vi "Assemble all modules.vi"(2 "Module List 2":T4(array[cluster])=[{"Enable"=TRUE, "Abs Start Time"="", "Module"=1, "String"="laser relock", "Array"=["A", "1"]}, {"Enable"=FALSE, "Abs Start Time"="", "Module"=0, "String"="", "Array"=["c", "7"]}, {"Enable"=TRUE, "Abs Start Time"="", "Module"=8, "String"="", "Array"=[]}, {"Enable"=TRUE, "Abs Start Time"="", "Module"=0, "String"="IP bias bleed on", "Array"=["B", "3"]}, {"Enable"=TRUE, "Abs Start Time"="", "Module"=0, "String"="IP master switch on", "Array"=["B", "2"]}, {"Enable"=FALSE, "Abs Start Time"="", "Module"=11, "String"="", "Array"=[]}, {"Enable"=FALSE, "Abs Start Time"="", "Module"=0, "String"="laser unlock for return", "Array"=["A", "1"]}, {"Enable"=FALSE, "Abs Start Time"="", "Module"=1, "String"="laser unlock for return", "Array"=["A", "1"]}, {"Enable"=FALSE, "Abs Start Time"="", "Module"=20, "String"="E/W shim for MOT", "Array"=["0", "0"]}, {"Enable"=FALSE, "Abs Start Time"="", "Module"=20, "String"="U/D shim for MOT", "Array"=["1", "-1"]}, {"Enable"=FALSE, "Abs Start Time"="", "Module"=20, "String"="N/S shim for MOT", "Array"=["2", "-1.5"]}, {"Enable"=FALSE, "Abs Start Time"="", "Module"=3, "String"="", "Array"=[]}] {"Module" items=["TTL high                                                                                 ", "TTL low                          ", "Camera Strobe                   ", "CMOT", "Defaults                           ", "Fluorescence pulse           ", "IP trap                         ", "Kinetics OD image          ", "Kinetics picture", "Kinetics probe pulse", "MOT light only                ", "MOT off                                   ", "MOT on                         ", "Move cart                      ", "OD image                     ", "Optical pumping          ", "Picture                             ", "Probe Pulse", "Quadrupole trap             ", "Quadrupole trap off", "QTrap off for OT        ", "Rb removal       ", "Molasses          ", "STIRAP", "OT B Field Off", "High field     ", "Utility Module 07     ", "Low Field", "Final B field ramps    ", "K removal    ", "Static DAC", "GPIB", "Molecule OD image", "Mol probe pulse", "Mol picture", "Unused OD image", "Unused probe pulse", "Unused picture", "K img repump", "STIRAP back 4 imaging", "B Field off", "Field Calibration", "Utility Module 15", "Utility Module 16", "Utility Module 17", "Utility Module 18", "Utility Module 19", "Utility Module 20"]}, 3 "durations":dbl[](array[numeric])=[0.0, 2400.0, 8635.078497322447, 3100.0, 1000.0, 2000.0] format="%.2f", 4 "Module List 6":T4(array[cluster])=[{"Enable"=TRUE, "Abs Start Time"="", "Module"=1, "String"="", "Array"=["c", "7"]}] {"Module" items=["TTL high                                                                                 ", "TTL low                          ", "Camera Strobe                   ", "CMOT", "Defaults                           ", "Fluorescence pulse           ", "IP trap                         ", "Kinetics OD image          ", "Kinetics picture", "Kinetics probe pulse", "MOT light only                ", "MOT off                                   ", "MOT on                         ", "Move cart                      ", "OD image                     ", "Optical pumping          ", "Picture                             ", "Probe Pulse", "Quadrupole trap             ", "Quadrupole trap off", "QTrap off for OT        ", "Rb removal       ", "Molasses          ", "STIRAP", "OT B Field Off", "High field     ", "Utility Module 07     ", "Low Field", "Final B field ramps    ", "K removal    ", "Static DAC", "GPIB", "Molecule OD image", "Mol probe pulse", "Mol picture", "Unused OD image", "Unused probe pulse", "Unused picture", "K img repump", "STIRAP back 4 imaging", "B Field off", "Field Calibration", "Utility Module 15", "Utility Module 16", "Utility Module 17", "Utility Module 18", "Utility Module 19", "Utility Module 20"]}, 5 "Module List 1":T4(array[cluster])=[{"Enable"=TRUE, "Abs Start Time"="", "Module"=0, "String"="dynamic DAC trigger", "Array"=["D", "14"]}, {"Enable"=TRUE, "Abs Start Time"="", "Module"=1, "String"="trigger down", "Array"=["D", "14"]}, {"Enable"=TRUE, "Abs Start Time"="", "Module"=19, "String"="", "Array"=[]}, {"Enable"=TRUE, "Abs Start Time"="", "Module"=20, "String"="K trap freq for CMOT", "Array"=["5", "4.6"]}, {"Enable"=TRUE, "Abs Start Time"="", "Module"=20, "String"="E/W shim for Qtrap loading", "Array"=["0", "-1"]}, {"Enable"=TRUE, "Abs Start Time"="", "Module"=20, "String"="U/D shim for Qtrap loading", "Array"=["1", "-1.5"]}, {"Enable"=TRUE, "Abs Start Time"="", "Module"=20, "String"="N/S shim for Qtrap loading", "Array"=["2", "-1"]}, {"Enable"=TRUE, "Abs Start Time"="", "Module"=20, "String"="repump K freq for OP", "Array"=["3", "0.05"]}, {"Enable"=TRUE, "Abs Start Time"="", "Module"=20, "String"="E/W shim for molasses 0", "Array"=["0", "-1"]}, {"Enable"=TRUE, "Abs Start Time"="", "Module"=20, "String"="U/D shim for molasses -0.6", "Array"=["1", "0.1"]}, {"Enable"=TRUE, "Abs Start Time"="", "Module"=20, "String"="N/S shim for molasses 0", "Array"=["2", "2"]}, {"Enable"=TRUE, "Abs Start Time"="", "Module"=8, "String"="", "Array"=["", ""]}, {"Enable"=TRUE, "Abs Start Time"="", "Module"=1, "String"="close Rb shutter(takes 1.4 ms", "Array"=["B", "0"]}, {"Enable"=FALSE, "Abs Start Time"="", "Module"=12, "String"="\n", "Array"=[]}, {"Enable"=FALSE, "Abs Start Time"="", "Module"=0, "String"="scope trigger", "Array"=["c", "7"]}, {"Enable"=FALSE, "Abs Start Time"="", "Module"=1, "String"="", "Array"=["c", "7"]}, {"Enable"=TRUE, "Abs Start Time"="", "Module"=14, "String"="", "Array"=[]}, {"Enable"=TRUE, "Abs Start Time"="", "Module"=20, "String"="K trap freq for MOT", "Array"=["5", "4.3"]}, {"Enable"=TRUE, "Abs Start Time"="", "Module"=20, "String"=" K repump freq for MOT freq", "Array"=["3", "0"]}, {"Enable"=TRUE, "Abs Start Time"="", "Module"=20, "String"="E/W shim for Qtrap", "Array"=["0", "2"]}, {"Enable"=TRUE, "Abs Start Time"="", "Module"=20, "String"="U/D shim for Qtrap", "Array"=["1", "2"]}, {"Enable"=TRUE, "Abs Start Time"="", "Module"=20, "String"="N/S shim for Qtrap", "Array"=["2", "2"]}, {"Enable"=TRUE, "Abs Start Time"="", "Module"=10, "String"="", "Array"=["-10"]}, {"Enable"=TRUE, "Abs Start Time"="", "Module"=0, "String"="laser unlock", "Array"=["A", "1"]}] {"Module" items=["TTL high                                                                                 ", "TTL low                          ", "Camera Strobe                   ", "CMOT", "Defaults                           ", "Fluorescence pulse           ", "IP trap                         ", "Kinetics OD image          ", "Kinetics picture", "Kinetics probe pulse", "MOT light only                ", "MOT off                                   ", "MOT on                         ", "Move cart                      ", "OD image                     ", "Optical pumping          ", "Picture                             ", "Probe Pulse", "Quadrupole trap             ", "Quadrupole trap off", "QTrap off for OT        ", "Rb removal       ", "Molasses          ", "STIRAP", "OT B Field Off", "High field     ", "Utility Module 07     ", "Low Field", "Final B field ramps    ", "K removal    ", "Static DAC", "GPIB", "Molecule OD image", "Mol probe pulse", "Mol picture", "Unused OD image", "Unused probe pulse", "Unused picture", "K img repump", "STIRAP back 4 imaging", "B Field off", "Field Calibration", "Utility Module 15", "Utility Module 16", "Utility Module 17", "Utility Module 18", "Utility Module 19", "Utility Module 20"]}, 6 "Module List 5":T4(array[cluster])=[{"Enable"=TRUE, "Abs Start Time"="", "Module"=0, "String"="", "Array"=["c", "7"]}] {"Module" items=["TTL high                                                                                 ", "TTL low                          ", "Camera Strobe                   ", "CMOT", "Defaults                           ", "Fluorescence pulse           ", "IP trap                         ", "Kinetics OD image          ", "Kinetics picture", "Kinetics probe pulse", "MOT light only                ", "MOT off                                   ", "MOT on                         ", "Move cart                      ", "OD image                     ", "Optical pumping          ", "Picture                             ", "Probe Pulse", "Quadrupole trap             ", "Quadrupole trap off", "QTrap off for OT        ", "Rb removal       ", "Molasses          ", "STIRAP", "OT B Field Off", "High field     ", "Utility Module 07     ", "Low Field", "Final B field ramps    ", "K removal    ", "Static DAC", "GPIB", "Molecule OD image", "Mol probe pulse", "Mol picture", "Unused OD image", "Unused probe pulse", "Unused picture", "K img repump", "STIRAP back 4 imaging", "B Field off", "Field Calibration", "Utility Module 15", "Utility Module 16", "Utility Module 17", "Utility Module 18", "Utility Module 19", "Utility Module 20"]}, 7 "Module List 4":T4(array[cluster])=[{"Enable"=TRUE, "Abs Start Time"="", "Module"=1, "String"="IP master switch off", "Array"=["B", "2"]}, {"Enable"=TRUE, "Abs Start Time"="", "Module"=0, "String"="trigger scope", "Array"=["c", "7"]}, {"Enable"=TRUE, "Abs Start Time"="", "Module"=11, "String"="", "Array"=[]}, {"Enable"=TRUE, "Abs Start Time"="", "Module"=0, "String"="laser unlock for cart return", "Array"=["A", "1"]}, {"Enable"=TRUE, "Abs Start Time"="", "Module"=1, "String"="laser relock", "Array"=["A", "1"]}, {"Enable"=TRUE, "Abs Start Time"="", "Module"=20, "String"="E/W shim for MOT", "Array"=["0", "0"]}, {"Enable"=TRUE, "Abs Start Time"="", "Module"=20, "String"="U/D shim for MOT", "Array"=["1", "-1"]}, {"Enable"=TRUE, "Abs Start Time"="", "Module"=20, "String"="N/S shim for MOT", "Array"=["2", "-1.5"]}, {"Enable"=TRUE, "Abs Start Time"="", "Module"=3, "String"="", "Array"=[]}, {"Enable"=FALSE, "Abs Start Time"="", "Module"=3, "String"="", "Array"=[]}] {"Module" items=["TTL high                                                                                 ", "TTL low                          ", "Camera Strobe                   ", "CMOT", "Defaults                           ", "Fluorescence pulse           ", "IP trap                         ", "Kinetics OD image          ", "Kinetics picture", "Kinetics probe pulse", "MOT light only                ", "MOT off                                   ", "MOT on                         ", "Move cart                      ", "OD image                     ", "Optical pumping          ", "Picture                             ", "Probe Pulse", "Quadrupole trap             ", "Quadrupole trap off", "QTrap off for OT        ", "Rb removal       ", "Molasses          ", "STIRAP", "OT B Field Off", "High field     ", "Utility Module 07     ", "Low Field", "Final B field ramps    ", "K removal    ", "Static DAC", "GPIB", "Molecule OD image", "Mol probe pulse", "Mol picture", "Unused OD image", "Unused probe pulse", "Unused picture", "K img repump", "STIRAP back 4 imaging", "B Field off", "Field Calibration", "Utility Module 15", "Utility Module 16", "Utility Module 17", "Utility Module 18", "Utility Module 19", "Utility Module 20"]}, 8 "Module List 3":T4(array[cluster])=[{"Enable"=FALSE, "Abs Start Time"="", "Module"=0, "String"="", "Array"=[]}] {"Module" items=["TTL high                                                                                 ", "TTL low                          ", "Camera Strobe                   ", "CMOT", "Defaults                           ", "Fluorescence pulse           ", "IP trap                         ", "Kinetics OD image          ", "Kinetics picture", "Kinetics probe pulse", "MOT light only                ", "MOT off                                   ", "MOT on                         ", "Move cart                      ", "OD image                     ", "Optical pumping          ", "Picture                             ", "Probe Pulse", "Quadrupole trap             ", "Quadrupole trap off", "QTrap off for OT        ", "Rb removal       ", "Molasses          ", "STIRAP", "OT B Field Off", "High field     ", "Utility Module 07     ", "Low Field", "Final B field ramps    ", "K removal    ", "Static DAC", "GPIB", "Molecule OD image", "Mol probe pulse", "Mol picture", "Unused OD image", "Unused probe pulse", "Unused picture", "K img repump", "STIRAP back 4 imaging", "B Field off", "Field Calibration", "Utility Module 15", "Utility Module 16", "Utility Module 17", "Utility Module 18", "Utility Module 19", "Utility Module 20"]}, 9 "Module Enabled Array":bool[](array[boolean])=[TRUE, TRUE, TRUE, TRUE, TRUE, TRUE]) -> (0 "Saveit Array":T2(array[cluster])=[{"Cluster"={"Enable"=TRUE, "Abs Start Time"=0.1, "Module"=0, "String"="dynamic DAC trigger", "Array"=["D", "14"]}, "Ring"=0}, {"Cluster"={"Enable"=TRUE, "Abs Start Time"=10.0, "Module"=1, "String"="trigger down", "Array"=["D", "14"]}, "Ring"=0}, {"Cluster"={"Enable"=TRUE, "Abs Start Time"=947.0, "Module"=19, "String"="", "Array"=[]}, "Ring"=0}, {"Cluster"={"Enable"=TRUE, "Abs Start Time"=947.0, "Module"=20, "String"="K trap freq for CMOT", "Array"=["5", "4.6"]}, "Ring"=0}, {"Cluster"={"Enable"=TRUE, "Abs Start Time"=947.0, "Module"=20, "String"="E/W shim for Qtrap loading", "Array"=["0", "-1"]}, "Ring"=0}, {"Cluster"={"Enable"=TRUE, "Abs Start Time"=947.0, "Module"=20, "String"="U/D shim for Qtrap loading", "Array"=["1", "-1.5"]}, "Ring"=0}, {"Cluster"={"Enable"=TRUE, "Abs Start Time"=947.0, "Module"=20, "String"="N/S shim for Qtrap loading", "Array"=["2", "-1"]}, "Ring"=0}, {"Cluster"={"Enable"=TRUE, "Abs Start Time"=947.0, "Module"=20, "String"="repump K freq for OP", "Array"=["3", "0.05"]}, "Ring"=0}, {"Cluster"={"Enable"=TRUE, "Abs Start Time"=994.5, "Module"=20, "String"="E/W shim for molasses 0", "Array"=["0", "-1"]}, "Ring"=0}, {"Cluster"={"Enable"=TRUE, "Abs Start Time"=994.5, "Module"=20, "String"="U/D shim for molasses -0.6", "Array"=["1", "0.1"]}, "Ring"=0}, {"Cluster"={"Enable"=TRUE, "Abs Start Time"=994.5, "Module"=20, "String"="N/S shim for molasses 0", "Array"=["2", "2"]}, "Ring"=0}, {"Cluster"={"Enable"=TRUE, "Abs Start Time"=995.5, "Module"=8, "String"="", "Array"=["", ""]}, "Ring"=0}, {"Cluster"={"Enable"=TRUE, "Abs Start Time"=997.1, "Module"=1, "String"="close Rb shutter(takes 1.4 ms", "Array"=["B", "0"]}, "Ring"=0}, {"Cluster"={"Enable"=FALSE, "Abs Start Time"=998.5, "Module"=12, "String"="\n", "Array"=[]}, "Ring"=0}, {"Cluster"={"Enable"=FALSE, "Abs Start Time"=998.5, "Module"=0, "String"="scope trigger", "Array"=["c", "7"]}, "Ring"=0}, {"Cluster"={"Enable"=FALSE, "Abs Start Time"=999.0, "Module"=1, "String"="", "Array"=["c", "7"]}, "Ring"=0}, {"Cluster"={"Enable"=TRUE, "Abs Start Time"=1000.0, "Module"=14, "String"="", "Array"=[]}, "Ring"=0}, {"Cluster"={"Enable"=TRUE, "Abs Start Time"=1000.0, "Module"=20, "String"="K trap freq for MOT", "Array"=["5", "4.3"]}, "Ring"=0}, {"Cluster"={"Enable"=TRUE, "Abs Start Time"=1000.0, "Module"=20, "String"=" K repump freq for MOT freq", "Array"=["3", "0"]}, "Ring"=0}, {"Cluster"={"Enable"=TRUE, "Abs Start Time"=1000.0, "Module"=20, "String"="E/W shim for Qtrap", "Array"=["0", "2"]}, "Ring"=0}, {"Cluster"={"Enable"=TRUE, "Abs Start Time"=1000.0, "Module"=20, "String"="U/D shim for Qtrap", "Array"=["1", "2"]}, "Ring"=0}, {"Cluster"={"Enable"=TRUE, "Abs Start Time"=1000.0, "Module"=20, "String"="N/S shim for Qtrap", "Array"=["2", "2"]}, "Ring"=0}, {"Cluster"={"Enable"=TRUE, "Abs Start Time"=1000.0, "Module"=10, "String"="", "Array"=["-10"]}, "Ring"=0}, {"Cluster"={"Enable"=TRUE, "Abs Start Time"=1000.0, "Module"=0, "String"="laser unlock", "Array"=["A", "1"]}, "Ring"=0}, {"Cluster"={"Enable"=TRUE, "Abs Start Time"=0.0, "Module"=1, "String"="laser relock", "Array"=["A", "1"]}, "Ring"=1}, {"Cluster"={"Enable"=FALSE, "Abs Start Time"=500.0, "Module"=0, "String"="", "Array"=["c", "7"]}, "Ring"=1}, {"Cluster"={"Enable"=TRUE, "Abs Start Time"=500.0, "Module"=8, "String"="", "Array"=[]}, "Ring"=1}, {"Cluster"={"Enable"=TRUE, "Abs Start Time"=400.0, "Module"=0, "String"="IP bias bleed on", "Array"=["B", "3"]}, "Ring"=1}, {"Cluster"={"Enable"=TRUE, "Abs Start Time"=500.0, "Module"=0, "String"="IP master switch on", "Array"=["B", "2"]}, "Ring"=1}, {"Cluster"={"Enable"=FALSE, "Abs Start Time"=505.0, "Module"=11, "String"="", "Array"=[]}, "Ring"=1}, {"Cluster"={"Enable"=FALSE, "Abs Start Time"=2000.0, "Module"=0, "String"="laser unlock for return", "Array"=["A", "1"]}, "Ring"=1}, {"Cluster"={"Enable"=FALSE, "Abs Start Time"=3500.0, "Module"=1, "String"="laser unlock for return", "Array"=["A", "1"]}, "Ring"=1}, {"Cluster"={"Enable"=FALSE, "Abs Start Time"=3600.0, "Module"=20, "String"="E/W shim for MOT", "Array"=["0", "0"]}, "Ring"=1}, {"Cluster"={"Enable"=FALSE, "Abs Start Time"=3600.0, "Module"=20, "String"="U/D shim for MOT", "Array"=["1", "-1"]}, "Ring"=1}, {"Cluster"={"Enable"=FALSE, "Abs Start Time"=3600.0, "Module"=20, "String"="N/S shim for MOT", "Array"=["2", "-1.5"]}, "Ring"=1}, {"Cluster"={"Enable"=FALSE, "Abs Start Time"=18500.0, "Module"=3, "String"="", "Array"=[]}, "Ring"=1}, {"Cluster"={"Enable"=FALSE, "Abs Start Time"=0.0, "Module"=0, "String"="", "Array"=[]}, "Ring"=2}, {"Cluster"={"Enable"=TRUE, "Abs Start Time"=0.0, "Module"=1, "String"="IP master switch off", "Array"=["B", "2"]}, "Ring"=3}, {"Cluster"={"Enable"=TRUE, "Abs Start Time"=0.0, "Module"=0, "String"="trigger scope", "Array"=["c", "7"]}, "Ring"=3}, {"Cluster"={"Enable"=TRUE, "Abs Start Time"=5.0, "Module"=11, "String"="", "Array"=[]}, "Ring"=3}, {"Cluster"={"Enable"=TRUE, "Abs Start Time"=1500.0, "Module"=0, "String"="laser unlock for cart return", "Array"=["A", "1"]}, "Ring"=3}, {"Cluster"={"Enable"=TRUE, "Abs Start Time"=3000.0, "Module"=1, "String"="laser relock", "Array"=["A", "1"]}, "Ring"=3}, {"Cluster"={"Enable"=TRUE, "Abs Start Time"=3000.0, "Module"=20, "String"="E/W shim for MOT", "Array"=["0", "0"]}, "Ring"=3}, {"Cluster"={"Enable"=TRUE, "Abs Start Time"=3000.0, "Module"=20, "String"="U/D shim for MOT", "Array"=["1", "-1"]}, "Ring"=3}, {"Cluster"={"Enable"=TRUE, "Abs Start Time"=3000.0, "Module"=20, "String"="N/S shim for MOT", "Array"=["2", "-1.5"]}, "Ring"=3}, {"Cluster"={"Enable"=TRUE, "Abs Start Time"=3100.0, "Module"=3, "String"="", "Array"=[]}, "Ring"=3}, {"Cluster"={"Enable"=FALSE, "Abs Start Time"=18000.0, "Module"=3, "String"="", "Array"=[]}, "Ring"=3}, {"Cluster"={"Enable"=TRUE, "Abs Start Time"=0.0, "Module"=0, "String"="", "Array"=["c", "7"]}, "Ring"=4}, {"Cluster"={"Enable"=TRUE, "Abs Start Time"=200.0, "Module"=1, "String"="", "Array"=["c", "7"]}, "Ring"=5}] {"Ring" items=["TTL high                                                                                 ", "TTL low                          ", "Camera Strobe                   ", "Defaults                           ", "Fluorescence pulse           ", "IP trap                         ", "Kinetics OD image          ", "MOT light only                ", "MOT off                                   ", "MOT on                         ", "Move cart                      ", "OD image                     ", "Optical pumping          ", "Picture                             ", "Quadrupole trap             ", "Utility Module 01          ", "Utility Module 02           ", "Utility Module 03           ", "Utility Module 04           ", "CMOT", "Static DAQ", "GPIB"]; "Cluster"."Module" items=["TTL high                                                                                 ", "TTL low                          ", "Camera Strobe                   ", "CMOT", "Defaults                           ", "Fluorescence pulse           ", "IP trap                         ", "Kinetics OD image          ", "Kinetics picture", "Kinetics probe pulse", "MOT light only                ", "MOT off                                   ", "MOT on                         ", "Move cart                      ", "OD image                     ", "Optical pumping          ", "Picture                             ", "Probe Pulse", "Quadrupole trap             ", "Quadrupole trap off", "QTrap off for OT        ", "Rb removal       ", "Molasses          ", "STIRAP", "OT B Field Off", "High field     ", "Utility Module 07     ", "Low Field", "Final B field ramps    ", "K removal    ", "Static DAC", "GPIB", "Molecule OD image", "Mol probe pulse", "Mol picture", "Unused OD image", "Unused probe pulse", "Unused picture", "K img repump", "STIRAP back 4 imaging", "B Field off", "Field Calibration", "Utility Module 15", "Utility Module 16", "Utility Module 17", "Utility Module 18", "Utility Module 19", "Utility Module 20"]; "Cluster"."Abs Start Time" format="%.3f"}, 1 "Module Array":T1(array[cluster])=[{"Enable"=TRUE, "Abs Start Time"=0.1, "Module"=0, "String"="dynamic DAC trigger", "Array"=["D", "14"]}, {"Enable"=TRUE, "Abs Start Time"=10.0, "Module"=1, "String"="trigger down", "Array"=["D", "14"]}, {"Enable"=TRUE, "Abs Start Time"=947.0, "Module"=19, "String"="", "Array"=[]}, {"Enable"=TRUE, "Abs Start Time"=947.0, "Module"=20, "String"="K trap freq for CMOT", "Array"=["5", "4.6"]}, {"Enable"=TRUE, "Abs Start Time"=947.0, "Module"=20, "String"="E/W shim for Qtrap loading", "Array"=["0", "-1"]}, {"Enable"=TRUE, "Abs Start Time"=947.0, "Module"=20, "String"="U/D shim for Qtrap loading", "Array"=["1", "-1.5"]}, {"Enable"=TRUE, "Abs Start Time"=947.0, "Module"=20, "String"="N/S shim for Qtrap loading", "Array"=["2", "-1"]}, {"Enable"=TRUE, "Abs Start Time"=947.0, "Module"=20, "String"="repump K freq for OP", "Array"=["3", "0.05"]}, {"Enable"=TRUE, "Abs Start Time"=994.5, "Module"=20, "String"="E/W shim for molasses 0", "Array"=["0", "-1"]}, {"Enable"=TRUE, "Abs Start Time"=994.5, "Module"=20, "String"="U/D shim for molasses -0.6", "Array"=["1", "0.1"]}, {"Enable"=TRUE, "Abs Start Time"=994.5, "Module"=20, "String"="N/S shim for molasses 0", "Array"=["2", "2"]}, {"Enable"=TRUE, "Abs Start Time"=995.5, "Module"=8, "String"="", "Array"=["", ""]}, {"Enable"=TRUE, "Abs Start Time"=997.1, "Module"=1, "String"="close Rb shutter(takes 1.4 ms", "Array"=["B", "0"]}, {"Enable"=FALSE, "Abs Start Time"=998.5, "Module"=12, "String"="\n", "Array"=[]}, {"Enable"=FALSE, "Abs Start Time"=998.5, "Module"=0, "String"="scope trigger", "Array"=["c", "7"]}, {"Enable"=FALSE, "Abs Start Time"=999.0, "Module"=1, "String"="", "Array"=["c", "7"]}, {"Enable"=TRUE, "Abs Start Time"=1000.0, "Module"=14, "String"="", "Array"=[]}, {"Enable"=TRUE, "Abs Start Time"=1000.0, "Module"=20, "String"="K trap freq for MOT", "Array"=["5", "4.3"]}, {"Enable"=TRUE, "Abs Start Time"=1000.0, "Module"=20, "String"=" K repump freq for MOT freq", "Array"=["3", "0"]}, {"Enable"=TRUE, "Abs Start Time"=1000.0, "Module"=20, "String"="E/W shim for Qtrap", "Array"=["0", "2"]}, {"Enable"=TRUE, "Abs Start Time"=1000.0, "Module"=20, "String"="U/D shim for Qtrap", "Array"=["1", "2"]}, {"Enable"=TRUE, "Abs Start Time"=1000.0, "Module"=20, "String"="N/S shim for Qtrap", "Array"=["2", "2"]}, {"Enable"=TRUE, "Abs Start Time"=1000.0, "Module"=10, "String"="", "Array"=["-10"]}, {"Enable"=TRUE, "Abs Start Time"=1000.0, "Module"=0, "String"="laser unlock", "Array"=["A", "1"]}, {"Enable"=TRUE, "Abs Start Time"=2400.0, "Module"=1, "String"="laser relock", "Array"=["A", "1"]}, {"Enable"=FALSE, "Abs Start Time"=2900.0, "Module"=0, "String"="", "Array"=["c", "7"]}, {"Enable"=TRUE, "Abs Start Time"=2900.0, "Module"=8, "String"="", "Array"=[]}, {"Enable"=TRUE, "Abs Start Time"=2800.0, "Module"=0, "String"="IP bias bleed on", "Array"=["B", "3"]}, {"Enable"=TRUE, "Abs Start Time"=2900.0, "Module"=0, "String"="IP master switch on", "Array"=["B", "2"]}, {"Enable"=FALSE, "Abs Start Time"=2905.0, "Module"=11, "String"="", "Array"=[]}, {"Enable"=FALSE, "Abs Start Time"=4400.0, "Module"=0, "String"="laser unlock for return", "Array"=["A", "1"]}, {"Enable"=FALSE, "Abs Start Time"=5900.0, "Module"=1, "String"="laser unlock for return", "Array"=["A", "1"]}, {"Enable"=FALSE, "Abs Start Time"=6000.0, "Module"=20, "String"="E/W shim for MOT", "Array"=["0", "0"]}, {"Enable"=FALSE, "Abs Start Time"=6000.0, "Module"=20, "String"="U/D shim for MOT", "Array"=["1", "-1"]}, {"Enable"=FALSE, "Abs Start Time"=6000.0, "Module"=20, "String"="N/S shim for MOT", "Array"=["2", "-1.5"]}, {"Enable"=FALSE, "Abs Start Time"=20900.0, "Module"=3, "String"="", "Array"=[]}, {"Enable"=FALSE, "Abs Start Time"=11035.078497322447, "Module"=0, "String"="", "Array"=[]}, {"Enable"=TRUE, "Abs Start Time"=14135.078497322447, "Module"=1, "String"="IP master switch off", "Array"=["B", "2"]}, {"Enable"=TRUE, "Abs Start Time"=14135.078497322447, "Module"=0, "String"="trigger scope", "Array"=["c", "7"]}, {"Enable"=TRUE, "Abs Start Time"=14140.078497322447, "Module"=11, "String"="", "Array"=[]}, {"Enable"=TRUE, "Abs Start Time"=15635.078497322447, "Module"=0, "String"="laser unlock for cart return", "Array"=["A", "1"]}, {"Enable"=TRUE, "Abs Start Time"=17135.078497322447, "Module"=1, "String"="laser relock", "Array"=["A", "1"]}, {"Enable"=TRUE, "Abs Start Time"=17135.078497322447, "Module"=20, "String"="E/W shim for MOT", "Array"=["0", "0"]}, {"Enable"=TRUE, "Abs Start Time"=17135.078497322447, "Module"=20, "String"="U/D shim for MOT", "Array"=["1", "-1"]}, {"Enable"=TRUE, "Abs Start Time"=17135.078497322447, "Module"=20, "String"="N/S shim for MOT", "Array"=["2", "-1.5"]}, {"Enable"=TRUE, "Abs Start Time"=17235.078497322447, "Module"=3, "String"="", "Array"=[]}, {"Enable"=FALSE, "Abs Start Time"=32135.078497322447, "Module"=3, "String"="", "Array"=[]}, {"Enable"=TRUE, "Abs Start Time"=15135.078497322447, "Module"=0, "String"="", "Array"=["c", "7"]}, {"Enable"=TRUE, "Abs Start Time"=17335.078497322447, "Module"=1, "String"="", "Array"=["c", "7"]}] {"Abs Start Time" format="%.2f"})   [LabVIEW 2017]
uses:
  globals/Modules global.vi
panel:
  in  "Tab Control":T3(tab)=enum."new stuff"
  # "This subVI assembles all six tabbed module lists into a single module array for output.  This array has all the relevant times from \"durations\" array added.  For the purposes of saving, there is a second output array called \"saveit array\"."
  # "Mot fill"
  # "Cart"
  # "Evap"
  # "Mag trap"
  # "Opt trap"
  # "New"
  # "After MOT fill"
  # "Enable  Time         Module                    Parameters                  Comments  \n                                                        (port A-D)   (line 0-15)"
  # "After cart transfer"
  # "Enable  Time         Module                    Parameters                  Comments  \n                                                        (port A-D)   (line 0-15)"
  # "After evaporation"
  # "Enable  Time         Module                    Parameters                  Comments  \n                                                        (port A-D)   (line 0-15)"
  # "After magnetic trap"
  # "Enable  Time         Module                    Parameters                  Comments  \n                                                        (port A-D)   (line 0-15)"
  # "After optical trap"
  # "Enable  Time         Module                    Parameters                  Comments  \n                                                        (port A-D)   (line 0-15)"
  # "new stuff"
  # "Enable  Time         Module                    Parameters                  Comments  \n                                                        (port A-D)   (line 0-15)"
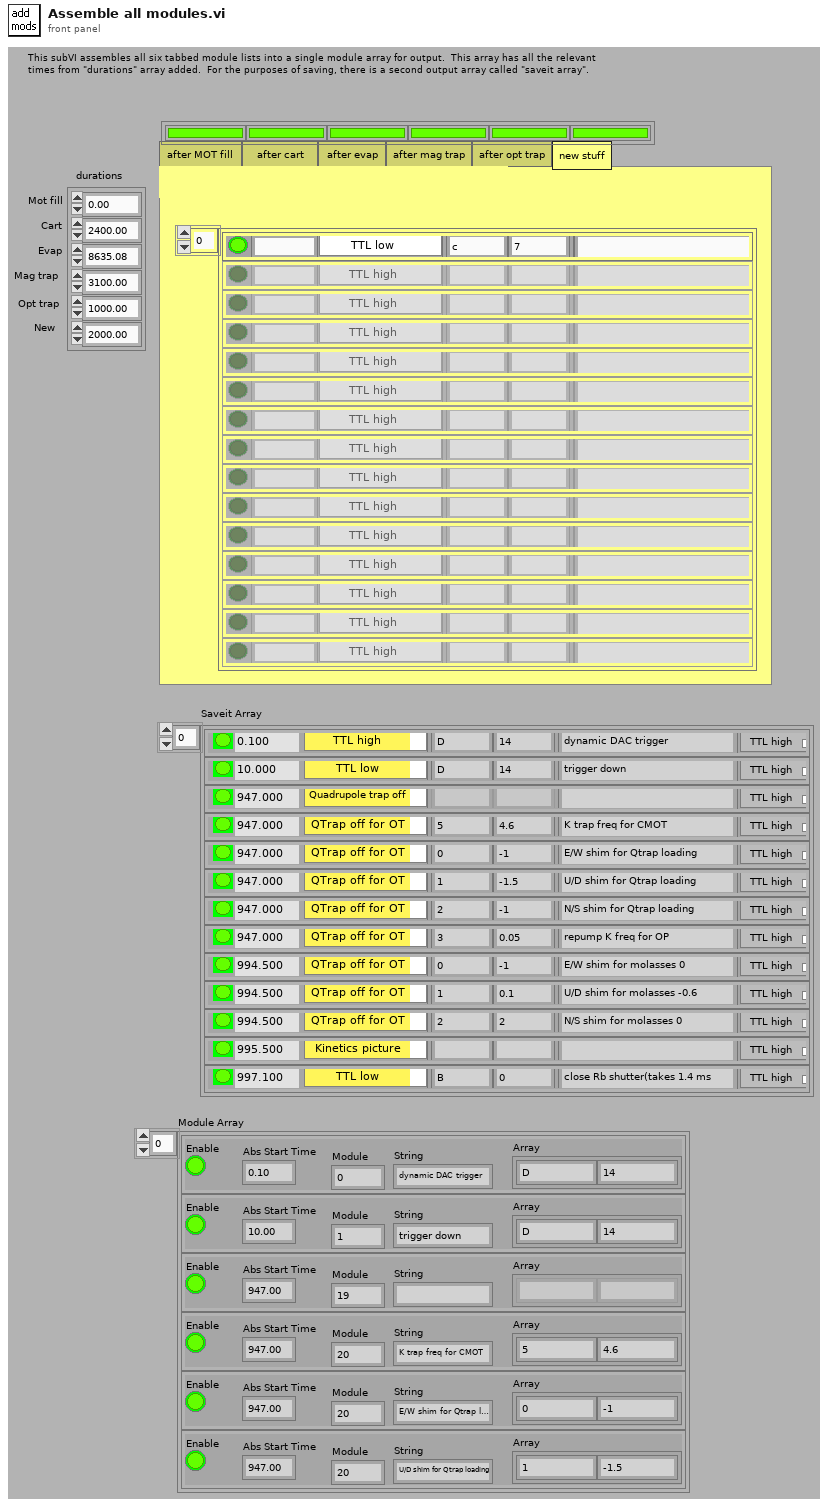
[diagram p1: front panel]
types:
  T1 = cluster{"Enable":bool, "Abs Start Time":dbl, "Module":u16, "String":string, "Array":string[]}[]
  T2 = cluster{"Cluster":cluster{"Enable":bool, "Abs Start Time":dbl, "Module":u16, "String":string, "Array":string[]}, "Ring":u16}[]
  T3 = enum32{"after MOT fill ", "after cart     ", "after evap ", "after mag trap", "after opt trap", "new stuff"}
  T4 = cluster{"Enable":bool, "Abs Start Time":string, "Module":u16, "String":string, "Array":string[]}[]
  T5 = cluster{"Cluster":cluster{"Enable":bool, "Abs Start Time":dbl, "Module":u16, "String":string, "Array":string[]}, "Element Data":u16}[]
  T6 = cluster{"Enable":bool, "Abs Start Time":dbl, "Module":u16, "String":string, "Array":string[]}
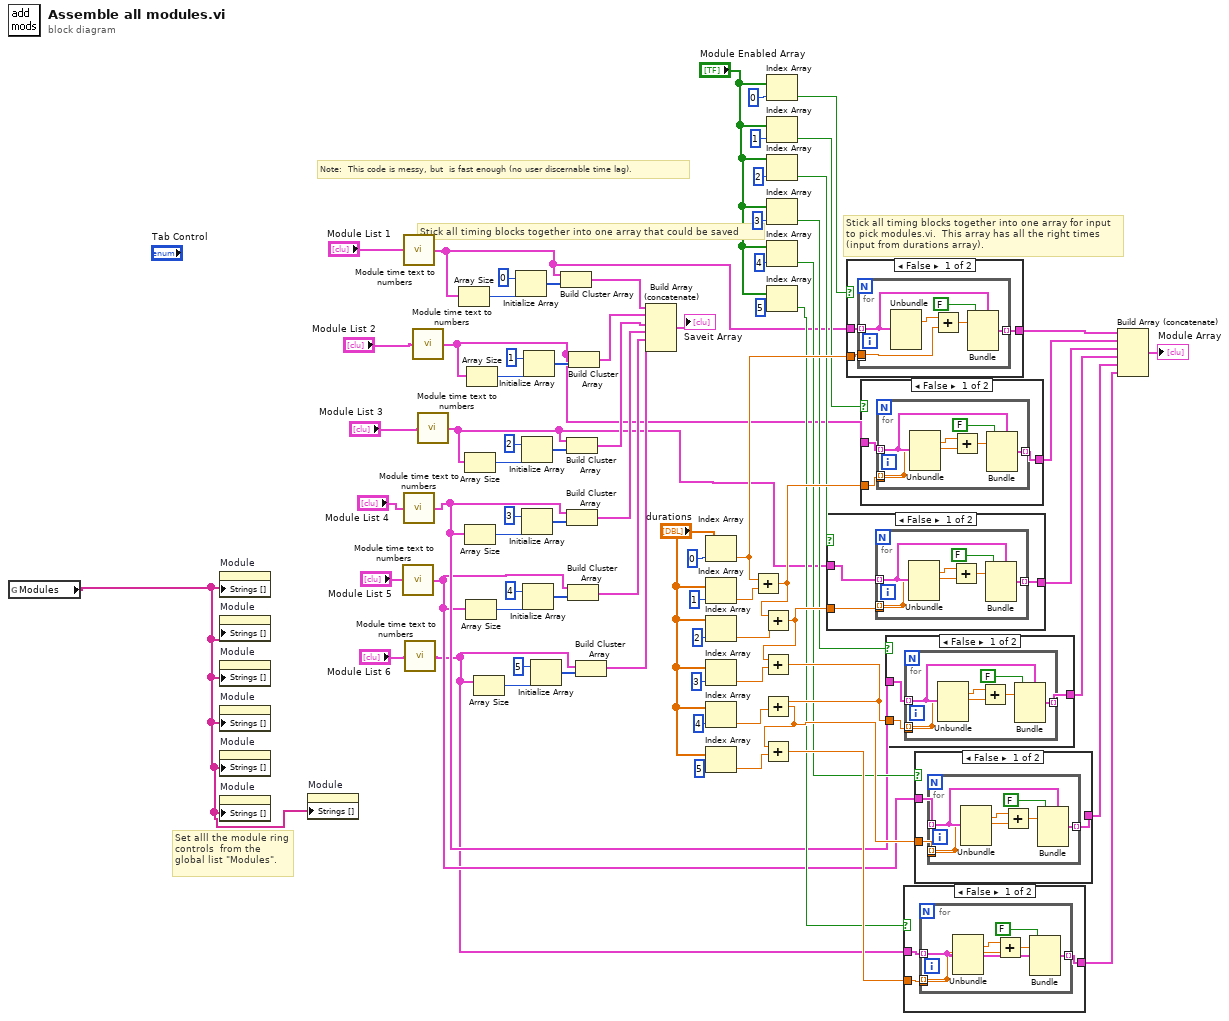
[diagram p0: block diagram]
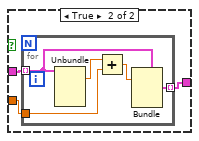
[diagram p2: hidden frame]
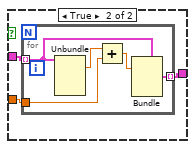
[diagram p3: hidden frame]
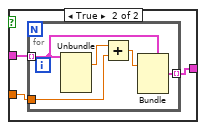
[diagram p4: hidden frame]
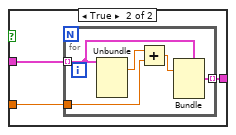
[diagram p5: hidden frame]
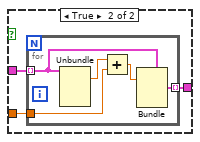
[diagram p6: hidden frame]
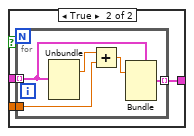
[diagram p7: hidden frame]
diagram:
  # "Stick all timing blocks together into one array for input to pick modules.vi.  This array has all the right times (input from durations array)."
  # "Note:  This code is messy, but  is fast enough (no user discernable time lag)."
  # "Set alll the module ring controls  from the global list \"Modules\"."
  # "Stick all timing blocks together into one array that could be saved"
  n1 = global read "Modules global.vi" "Modules"() -> (w13:string[])
  n2 = property on="Module" class="Ring (strict)"("Strings []"=w13) -> ()  [unwired: 2 in, 2 out]
  n3 = property on="Module" class="Ring (strict)"("Strings []"=w13) -> ()  [unwired: 2 in, 2 out]
  n4 = property on="Module" class="Ring (strict)"("Strings []"=w13) -> ()  [unwired: 2 in, 2 out]
  n5 = property on="Module" class="Ring (strict)"("Strings []"=w13) -> ()  [unwired: 2 in, 2 out]
  n6 = property on="Module" class="Ring (strict)"("Strings []"=w13) -> ()  [unwired: 2 in, 2 out]
  n7 = property on="Module" class="Ring (strict)"("Strings []"=w13) -> ()  [unwired: 2 in, 2 out]
  n8 = property on="Module" class="Ring (strict)"("Strings []"=w13) -> ()  [unwired: 2 in, 2 out]
  n9 = call "Module time text to numbers.vi"("Module List Text"="Module List 5") -> ("Module List Numbers"=w4:T1)
  n10 = call "Module time text to numbers.vi"("Module List Text"="Module List 1") -> ("Module List Numbers"=w12:T1)
  n11 = call "Module time text to numbers.vi"("Module List Text"="Module List 4") -> ("Module List Numbers"=w6:T1)
  n12 = call "Module time text to numbers.vi"("Module List Text"="Module List 6") -> ("Module List Numbers"=w1:T1)
  n13 = call "Module time text to numbers.vi"("Module List Text"="Module List 2") -> ("Module List Numbers"=w10:T1)
  n14 = call "Module time text to numbers.vi"("Module List Text"="Module List 3") -> ("Module List Numbers"=w7:T1)
  n15 = Array Size(array=w12) -> (size(s)=w75:i32)
  n16 = Array Size(array=w7) -> (size(s)=w67:i32)
  n17 = Array Size(array=w6) -> (size(s)=w63:i32)
  n18 = Array Size(array=w4) -> (size(s)=w60:i32)
  n19 = Array Size(array=w10) -> (size(s)=w71:i32)
  n20 = Array Size(array=w1) -> (size(s)=w55:i32)
  n21 = Initialize Array(u16 0 ("Element Data"), w75) -> (w74:u16[])
  n22 = Initialize Array(u16 2 ("Element Data"), w67) -> (w66:u16[])
  n23 = Initialize Array(u16 3 ("Element Data"), w63) -> (w62:u16[])
  n24 = Initialize Array(u16 4 ("Element Data"), w60) -> (w59:u16[])
  n25 = Initialize Array(u16 1 ("Element Data"), w71) -> (w70:u16[])
  n26 = Initialize Array(u16 5 ("Element Data"), w55) -> (w54:u16[])
  n27 = Build Cluster Array(w12, w74) -> (w73:T5)
  n28 = Build Cluster Array(w7, w66) -> (w65:T5)
  n29 = Build Cluster Array(w6, w62) -> (w58:T5)
  n30 = Build Cluster Array(w4, w59) -> (w57:T5)
  n31 = Build Cluster Array(w10, w70) -> (w69:T5)
  n32 = Build Cluster Array(w1, w54) -> (w52:T5)
  n33 = Build Array (concatenate)(w73, w69, w65, w58, w57, w52) -> (→"Saveit Array":T5)
  n34 = Index Array(array="durations", index=0 ("Index")) -> (element=w48:dbl)
  n35 = Index Array(array="durations", index=1 ("Index")) -> (element=w49:dbl)
  n36 = Index Array(array="durations", index=2 ("Index")) -> (element=w46:dbl)
  n37 = Index Array(array="durations", index=3 ("Index")) -> (element=w44:dbl)
  n38 = Index Array(array="durations", index=4 ("Index")) -> (element=w42:dbl)
  n39 = Index Array(array="durations", index=5 ("Index")) -> (element=w40:dbl)
  n40 = Add(x=w48, y=w49) -> (x+y=w37:dbl)
  n41 = Add(x=w37, y=w46) -> (x+y=w36:dbl)
  n42 = Add(x=w36, y=w44) -> (x+y=w35:dbl)
  n43 = Add(x=w35, y=w42) -> (x+y=w34:dbl)
  n44 = Add(x=w34, y=w40) -> (x+y=w33:dbl)
  n45 = Index Array(array="Module Enabled Array", index=0 ("Index")) -> (element=w20:bool)
  n46 = Index Array(array="Module Enabled Array", index=1 ("Index")) -> (element=w19:bool)
  n47 = Index Array(array="Module Enabled Array", index=2 ("Index")) -> (element=w18:bool)
  n48 = Index Array(array="Module Enabled Array", index=3 ("Index")) -> (element=w17:bool)
  n49 = Index Array(array="Module Enabled Array", index=4 ("Index")) -> (element=w16:bool)
  n50 = Index Array(array="Module Enabled Array", index=5 ("Index")) -> (element=w15:bool)
  n51 = case shown="False" w18 {
    tunnel: w36 -> [w78 w88]
    tunnel: [w77 w87] -> w27
    tunnel: w7 -> [w79 w86]
    frame False {
      n52 = for {
        tunnel: w79 -> [w84] mode=indexing
        tunnel: w78 -> [w81]
        tunnel: [w82] -> w77 mode=indexing
        tunnel: [w81] -> _ mode=indexing
        n53 = Unbundle(w84) -> ("Abs Start Time"=w85:dbl)  [unwired: 4 out]
        n54 = Add(x=w85, y=w81) -> (x+y=w83:dbl)
        n55 = Bundle(cluster=w84, "Enable"=FALSE, "Abs Start Time"=w83) -> (w82:T6)  [unwired: 3 in]
      }
    }
    frame True {
      n56 = for {
        tunnel: w86 -> [w92] mode=indexing
        tunnel: w88 -> [w93]
        tunnel: [w91] -> w87 mode=indexing
        n57 = Unbundle(w92) -> ("Abs Start Time"=w90:dbl)  [unwired: 4 out]
        n58 = Add(x=w90, y=w93) -> (x+y=w89:dbl)
        n59 = Bundle(cluster=w92, "Abs Start Time"=w89) -> (w91:T6)  [unwired: 4 in]
      }
    }
  }
  n60 = case shown="False" w20 {
    tunnel: w48 -> [w95 w105]
    tunnel: [w94 w104] -> w38
    tunnel: w12 -> [w96 w103]
    frame False {
      n61 = for {
        tunnel: w96 -> [w101] mode=indexing
        tunnel: [w98] -> _ mode=indexing
        tunnel: [w99] -> w94 mode=indexing
        tunnel: w95 -> [w98]
        n62 = Unbundle(w101) -> ("Abs Start Time"=w102:dbl)  [unwired: 4 out]
        n63 = Add(x=w102, y=w98) -> (x+y=w100:dbl)
        n64 = Bundle(cluster=w101, "Enable"=FALSE, "Abs Start Time"=w100) -> (w99:T6)  [unwired: 3 in]
      }
    }
    frame True {
      n65 = for {
        tunnel: w103 -> [w108] mode=indexing
        tunnel: w105 -> [w110]
        tunnel: [w106] -> w104 mode=indexing
        n66 = Unbundle(w108) -> ("Abs Start Time"=w109:dbl)  [unwired: 4 out]
        n67 = Add(x=w109, y=w110) -> (x+y=w107:dbl)
        n68 = Bundle(cluster=w108, "Abs Start Time"=w107) -> (w106:T6)  [unwired: 4 in]
      }
    }
  }
  n69 = case shown="False" w19 {
    tunnel: w37 -> [w111 w122]
    tunnel: [w112 w121] -> w28
    tunnel: w10 -> [w113 w120]
    frame False {
      n70 = for {
        tunnel: w113 -> [w118] mode=indexing
        tunnel: w111 -> [w115]
        tunnel: [w116] -> w112 mode=indexing
        tunnel: [w115] -> _ mode=indexing
        n71 = Unbundle(w118) -> ("Abs Start Time"=w119:dbl)  [unwired: 4 out]
        n72 = Add(x=w119, y=w115) -> (x+y=w117:dbl)
        n73 = Bundle(cluster=w118, "Enable"=FALSE, "Abs Start Time"=w117) -> (w116:T6)  [unwired: 3 in]
      }
    }
    frame True {
      n74 = for {
        tunnel: w120 -> [w126] mode=indexing
        tunnel: w122 -> [w127]
        tunnel: [w125] -> w121 mode=indexing
        n75 = Unbundle(w126) -> ("Abs Start Time"=w124:dbl)  [unwired: 4 out]
        n76 = Add(x=w124, y=w127) -> (x+y=w123:dbl)
        n77 = Bundle(cluster=w126, "Abs Start Time"=w123) -> (w125:T6)  [unwired: 4 in]
      }
    }
  }
  n78 = case shown="False" w17 {
    tunnel: w35 -> [w128 w139]
    tunnel: [w130 w138] -> w32
    tunnel: w6 -> [w129 w137]
    frame False {
      n79 = for {
        tunnel: w129 -> [w135] mode=indexing
        tunnel: w128 -> [w132]
        tunnel: [w133] -> w130 mode=indexing
        tunnel: [w132] -> _ mode=indexing
        n80 = Unbundle(w135) -> ("Abs Start Time"=w136:dbl)  [unwired: 4 out]
        n81 = Add(x=w136, y=w132) -> (x+y=w134:dbl)
        n82 = Bundle(cluster=w135, "Enable"=FALSE, "Abs Start Time"=w134) -> (w133:T6)  [unwired: 3 in]
      }
    }
    frame True {
      n83 = for {
        tunnel: w137 -> [w142] mode=indexing
        tunnel: w139 -> [w144]
        tunnel: [w140] -> w138 mode=indexing
        n84 = Unbundle(w142) -> ("Abs Start Time"=w143:dbl)  [unwired: 4 out]
        n85 = Add(x=w143, y=w144) -> (x+y=w141:dbl)
        n86 = Bundle(cluster=w142, "Abs Start Time"=w141) -> (w140:T6)  [unwired: 4 in]
      }
    }
  }
  n87 = case shown="False" w15 {
    tunnel: w33 -> [w146 w156]
    tunnel: [w145 w155] -> w30
    tunnel: w1 -> [w147 w154]
    frame False {
      n88 = for {
        tunnel: [w148] -> _ mode=indexing
        tunnel: w146 -> [w150]
        tunnel: [w151] -> w145 mode=indexing
        tunnel: [w150] -> _ mode=indexing
        tunnel: w147 -> [w148] mode=indexing
        n89 = Unbundle(w148) -> ("Abs Start Time"=w153:dbl)  [unwired: 4 out]
        n90 = Add(x=w153, y=w150) -> (x+y=w152:dbl)
        n91 = Bundle(cluster=w148, "Enable"=FALSE, "Abs Start Time"=w152) -> (w151:T6)  [unwired: 3 in]
      }
    }
    frame True {
      n92 = for {
        tunnel: w154 -> [w159] mode=indexing
        tunnel: w156 -> [w161]
        tunnel: [w157] -> w155 mode=indexing
        n93 = Unbundle(w159) -> ("Abs Start Time"=w160:dbl)  [unwired: 4 out]
        n94 = Add(x=w160, y=w161) -> (x+y=w158:dbl)
        n95 = Bundle(cluster=w159, "Abs Start Time"=w158) -> (w157:T6)  [unwired: 4 in]
      }
    }
  }
  n96 = case shown="False" w16 {
    tunnel: w34 -> [w164 w173]
    tunnel: [w162 w172] -> w31
    tunnel: w4 -> [w163 w171]
    frame False {
      n97 = for {
        tunnel: w163 -> [w169] mode=indexing
        tunnel: w164 -> [w166]
        tunnel: [w167] -> w162 mode=indexing
        tunnel: [w166] -> _ mode=indexing
        n98 = Unbundle(w169) -> ("Abs Start Time"=w170:dbl)  [unwired: 4 out]
        n99 = Add(x=w170, y=w166) -> (x+y=w168:dbl)
        n100 = Bundle(cluster=w169, "Enable"=FALSE, "Abs Start Time"=w168) -> (w167:T6)  [unwired: 3 in]
      }
    }
    frame True {
      n101 = for {
        tunnel: w171 -> [w176] mode=indexing
        tunnel: w173 -> [w178]
        tunnel: [w174] -> w172 mode=indexing
        n102 = Unbundle(w176) -> ("Abs Start Time"=w177:dbl)  [unwired: 4 out]
        n103 = Add(x=w177, y=w178) -> (x+y=w175:dbl)
        n104 = Bundle(cluster=w176, "Abs Start Time"=w175) -> (w174:T6)  [unwired: 4 in]
      }
    }
  }
  n105 = Build Array (concatenate)(w38, w28, w27, w32, w31, w30) -> (→"Module Array":T1)
